vi "EG_G5210 SetOscPar.vi"(6 "Amplitude(mV rms)":i32=2000 min=0 max=2000 step=1, 7 "Frequency":dbl=10000.0 min=0.5 max=120000.0 step=0.1, 8 "error in (no error)":errorcluster, 9 "Set to 5Vrms":bool, 10 "Énum":enum16{"Amplitude", "Frequency"}(ring), 11 "Ressource VISA":refnum<visa-resource-name>="GPIB0::8::INSTR") -> (0 "error out":errorcluster, 3 "Ressource VISA Out":refnum<visa-resource-name>="GPIB0::8::INSTR")   [LabVIEW 2010]
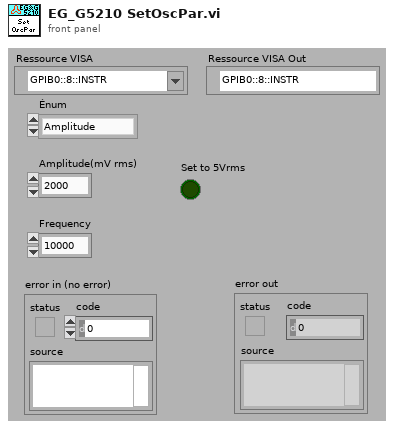
[diagram p1: front panel]
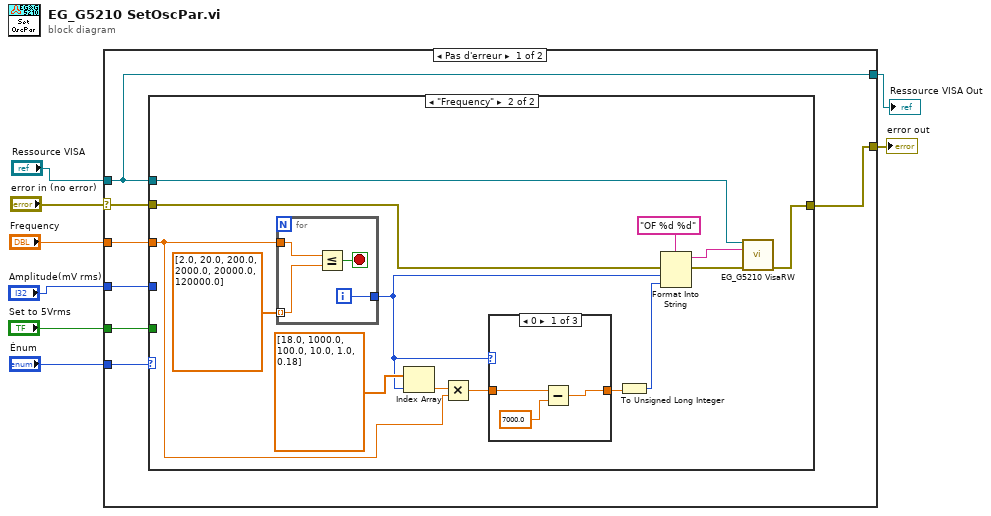
[diagram p0: block diagram]
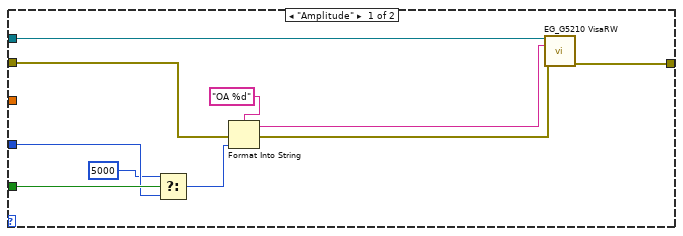
[diagram p2: hidden frame]
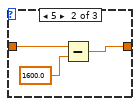
[diagram p3: hidden frame]
diagram:
  n1 = case shown="Pas d'erreur" "error in (no error)" {
    selector: "error in (no error)" -> [w14 w52]
    tunnel: [w15 w52] -> w7
    tunnel: [w13 w51] -> w6
    tunnel: "Ressource VISA" -> [w13 w51]
    tunnel: "Frequency" -> [w12 _]
    tunnel: "Énum" -> [w11 _]
    tunnel: "Amplitude(mV rms)" -> [w10 _]
    tunnel: "Set to 5Vrms" -> [w9 _]
    frame No Error {
      n2 = case shown="\"Frequency\"" w11 {
        tunnel: w14 -> [w21 w28]
        tunnel: [w25 w37] -> w15
        tunnel: w13 -> [w24 w39]
        tunnel: w12 -> [_ w35]
        tunnel: w10 -> [w18 _]
        tunnel: w9 -> [w19 _]
        frame "Amplitude" {
          n3 = Select(t=5000 ("cas vrai"), s=w19, f=w18) -> (s? t:f=w16:i32)
          n4 = Format Into String(format string="OA %d" ("ChaineCom"), error in=w21, w16) -> (resulting string=w22:string, error out=w20:errorcluster)  [unwired: 1 in]
          n5 = call <userlib>:"EG_G5210 VisaRW.vi"("VISA Rsrc"=w24, "ChaineCom"=w22, "error in (no error)"=w20) -> ("error out"=w25:errorcluster)  [unwired: 9 in, 3 out]
        }
        frame "Frequency" {
          n6 = for {
            tunnel: dbl[] [2.0, 20.0, 200.0, 2000.0, 20000.0, 120000.0] -> [w49] mode=indexing
            tunnel: w35 -> [w47]
            tunnel: [w48] -> w33
            i -> [w48]
            stop <- w50 stop-if-true
            n7 = Less Or Equal?(x=w47, y=w49) -> (x <= y?=w50:bool)
          }
          n8 = Index Array(array=dbl[] [18.0, 1000.0, 100.0, 10.0, 1.0, 0.18], index=w33) -> (element=w34:dbl)
          n9 = Multiply(x=w34, y=w35) -> (x*y=w32:dbl)
          n10 = case shown="0" w33 {
            tunnel: w32 -> [w41 w44 w46]
            tunnel: [w40 w43 w46] -> w31
            frame 0 {
              n11 = Subtract(x=w41, y=7000.0) -> (x-y=w40:dbl)
            }
            frame 5 {
              n12 = Subtract(x=w44, y=1600.0) -> (x-y=w43:dbl)
            }
            frame 1, Default {
            }
          }
          n13 = To Unsigned Long Integer(number=w31) -> (unsigned 32bit integer=w30:u32)
          n14 = Format Into String(format string="OF %d %d" ("ChaineCom"), error in=w28, w33, w30) -> (resulting string=w27:string, error out=w26:errorcluster)  [unwired: 1 in]
          n15 = call <userlib>:"EG_G5210 VisaRW.vi"("VISA Rsrc"=w39, "ChaineCom"=w27, "error in (no error)"=w26) -> ("error out"=w37:errorcluster)  [unwired: 9 in, 3 out]
        }
      }
    }
    frame Error {
    }
  }
  "error out" <- w7
  "Ressource VISA Out" <- w6
